vi "Create TDMS Log.vi"(8 "error in (no error)":errorcluster, 11 "Fault Index":i32) -> (0 "error out":errorcluster, 3 "Refnum out":refnum<k34>)   [LabVIEW 2014]
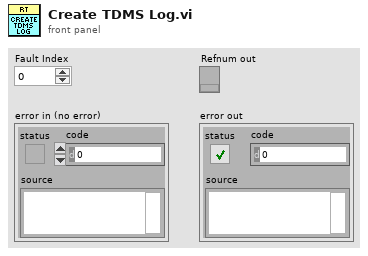
[diagram p1: front panel]
types:
  T1 = enum16{"open", "open or create", "create or replace", "create", "open (read-only)"}
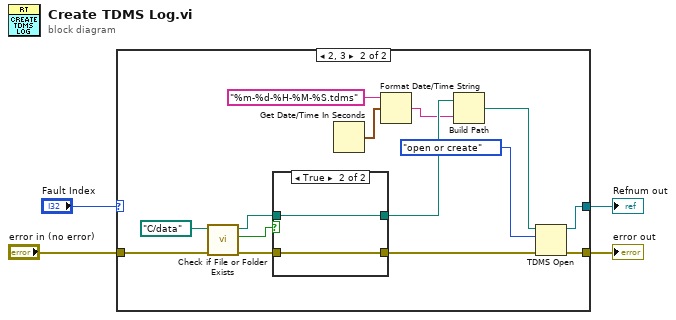
[diagram p0: block diagram]
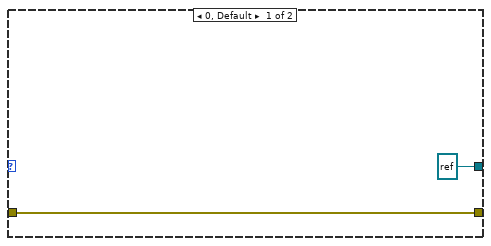
[diagram p2: hidden frame]
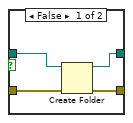
[diagram p3: hidden frame]
diagram:
  n1 = case shown="2, 3" "Fault Index" {
    tunnel: [refnum<k34> refnum ("tdms file out") w10] -> w4
    tunnel: [w5 w9] -> w3
    tunnel: "error in (no error)" -> [w5 w8]
    frame 0, Default {
    }
    frame 2, 3 {
      n2 = call <vilib>:"Check if File or Folder Exists.vi"("error in (no error)"=w8, "path"=path "C:/data") -> ("error out"=w12:errorcluster, "file or folder exists?"=w19:bool, "dup path"=w18:path)  [unwired: 7 in]
      n3 = case shown="True" w19 {
        tunnel: w18 -> [w24 w26]
        tunnel: [w23 w26] -> w17
        tunnel: w12 -> [w22 w25]
        tunnel: [w21 w25] -> w11
        frame False {
          n4 = Create Folder(path (use dialog)=w24, error in=w22) -> (created path=w23:path, error out=w21:errorcluster)  [unwired: 1 in, 1 out]
        }
        frame True {
        }
      }
      n5 = Get Date/Time In Seconds() -> (seconds since 1Jan1904=w16:timestamp)
      n6 = Format Date/Time String(time format string (%c)="%m-%d-%H-%M-%S.tdms", seconds (now)=w16) -> (date/time string=w14:string)  [unwired: 1 in]
      n7 = Build Path(base path=w17, name or relative path=w14) -> (appended path=w13:path)
      n8 = TDMS Open(8:w11, 10:T1."open or create" ("operation (0:open)"), 11:w13) -> (0:w9:errorcluster, 3:w10:refnum<k34>)  [unwired: 4 in]
    }
  }
  "error out" <- w3
  "Refnum out" <- w4
